vi "Read Laser Status.vi"(8 "error in (no error)":errorcluster, 11 "Laser Controller in":refnum<class "Laser Controller.lvclass">) -> (0 "error out":errorcluster, 2 "Process State Data":refnum<data-value>, 3 "Laser Controller out":refnum<class "Laser Controller.lvclass">)   [LabVIEW 2022 SP3, in "Laser Controller.lvclass"]
uses:
  Laser Controller.lvclass
  Laser Controller.lvclass/Laser Controller.ctl
  XY Stage/Process Actor/Process Framework/Process State Data/Process State Data.lvclass
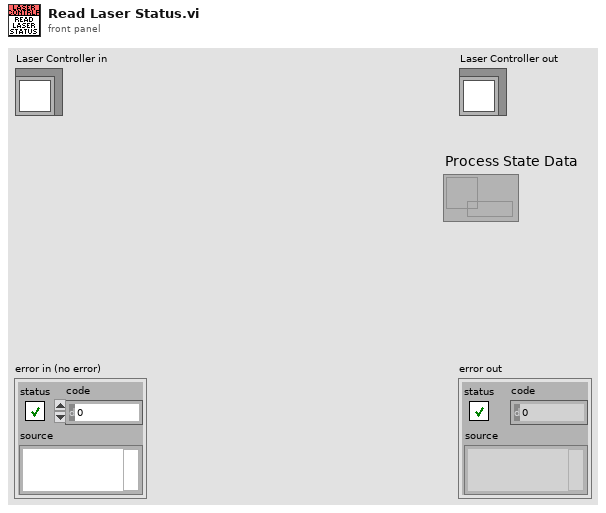
[diagram p1: front panel]
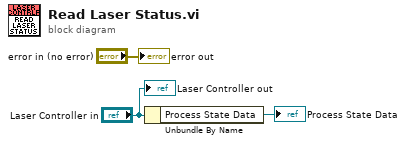
[diagram p0: block diagram]
diagram:
  n1 = Unbundle By Name("Laser Controller in") -> ("Process State Data"=→"Process State Data":refnum<data-value>)
  "error out" <- "error in (no error)"
  "Laser Controller out" <- "Laser Controller in"
